vi "Read Master Timing Module.vi"(8 "error in":errorcluster, 11 "Standard Engine Repo Data in":refnum<class "Standard Engine Configuration.lvclass">) -> (0 "error out":errorcluster, 2 "Master Timing Module":string, 3 "Standard Engine Repo Data out":refnum<class "Standard Engine Configuration.lvclass">)   [LabVIEW 2013, in "Standard Engine Configuration.lvclass"]
uses:
  Standard Engine Configuration.lvclass
  Standard Engine Configuration.lvclass/Standard Engine Configuration.ctl
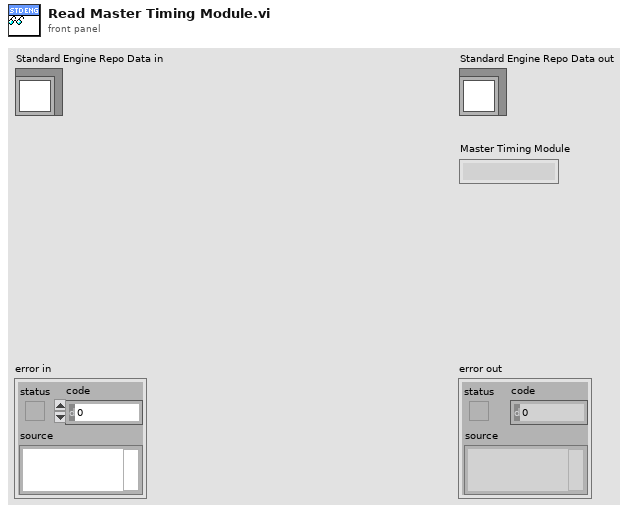
[diagram p1: front panel]
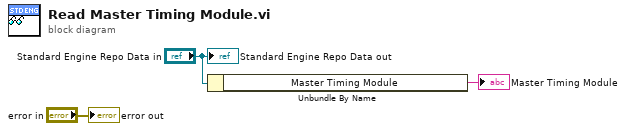
[diagram p0: block diagram]
diagram:
  n1 = Unbundle By Name("Standard Engine Repo Data in") -> ("Master Timing Module"=→"Master Timing Module":string)
  "error out" <- "error in"
  "Standard Engine Repo Data out" <- "Standard Engine Repo Data in"
